vi "_RT_CtrlLoop_Pub_Wfm_ProcessCodes.vi"(7 "Function":T1, 8 "error in (no error)":errorcluster, 10 "EventCodes_U64Arr in":u64[](array[numeric])) -> (0 "error out":errorcluster, 1 "SigLength out":i32, 2 "EventCodes_U64Arr out":u64[](array[numeric]), 4 "DynamicTimeout":i32)   [LabVIEW 2018]
uses:
  Ctl/_ctl_Integrated_Cmd.ctl
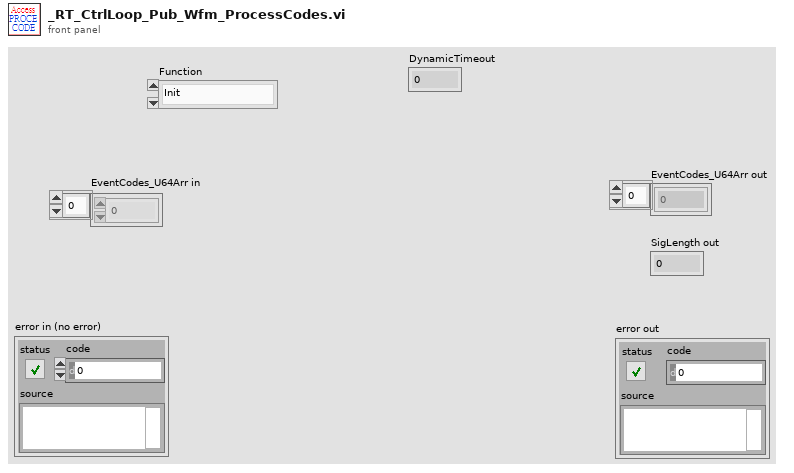
[diagram p1: front panel]
types:
  T1 = typedef "_ctl_Integrated_Cmd.ctl" = enum8{"Init", "Set", "Get", "Read", "Write", "Send", "Idle", "Startup", "Execution", "End", "Close"}
  T2 = enum16{"open", "replace", "create", "open or create", "replace or create", "replace or create with confirmation"}
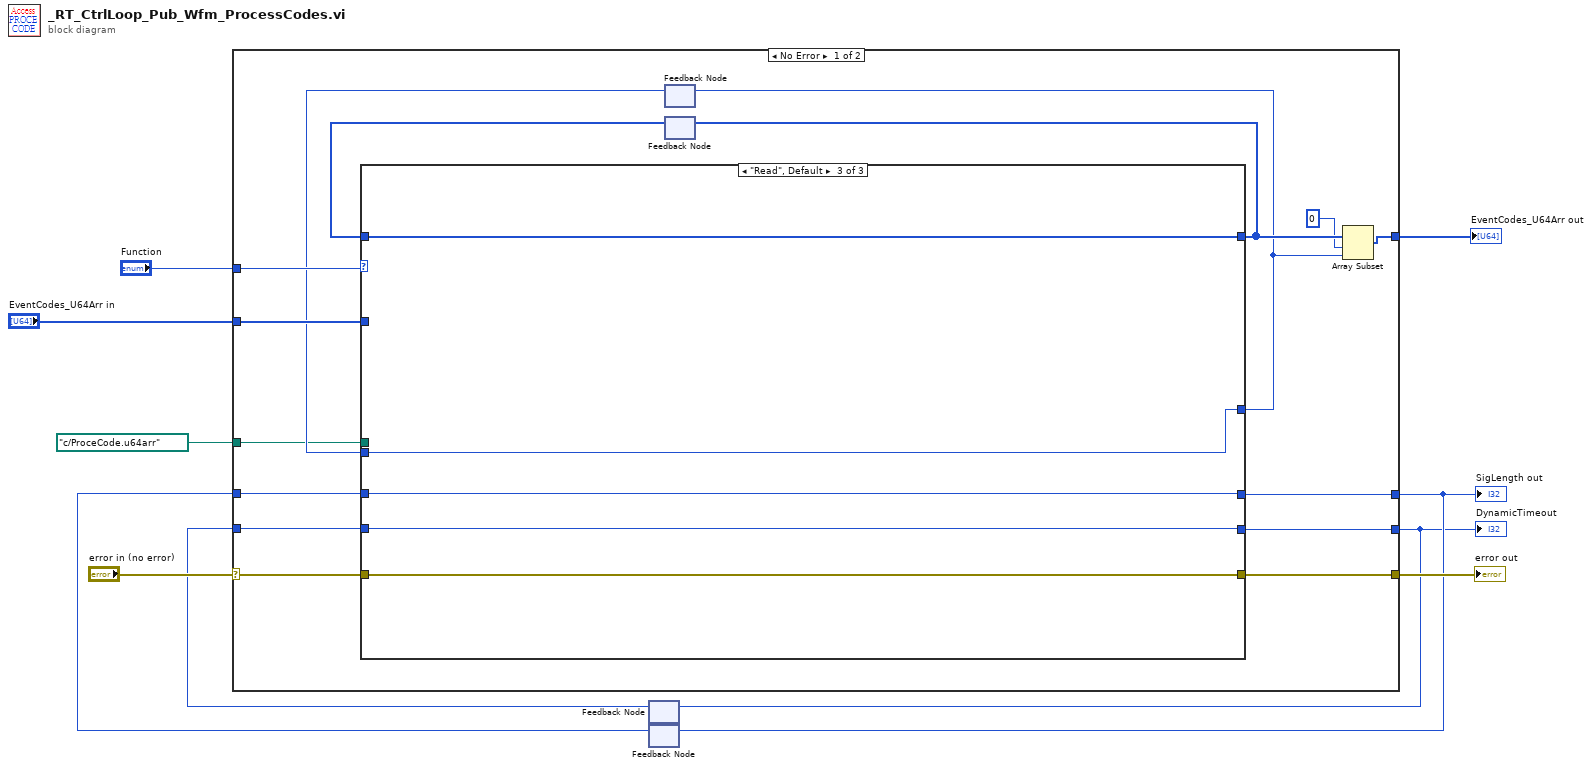
[diagram p0: block diagram]
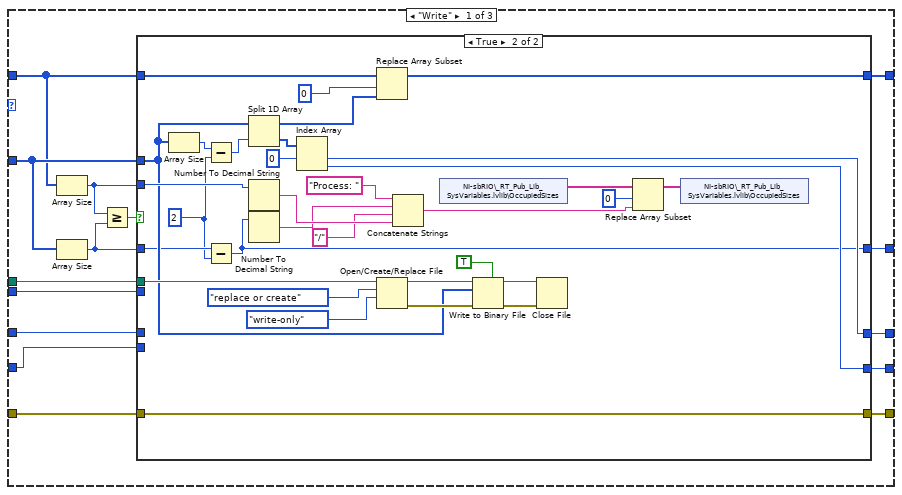
[diagram p2: hidden frame]
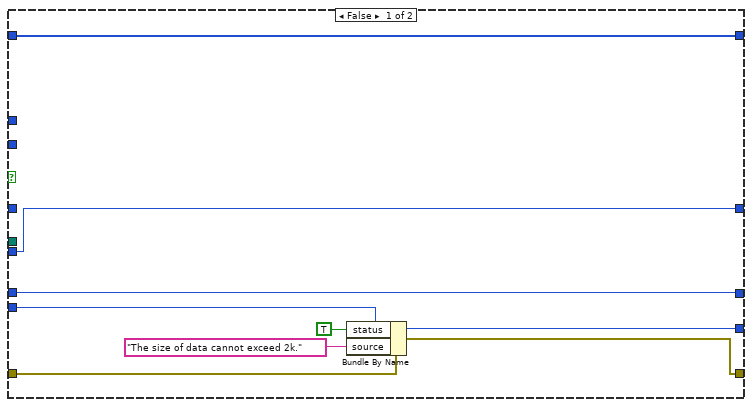
[diagram p3: hidden frame]
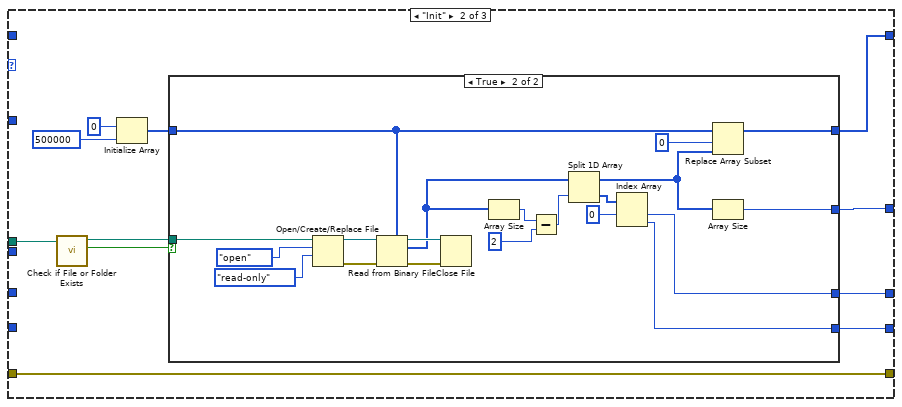
[diagram p4: hidden frame]
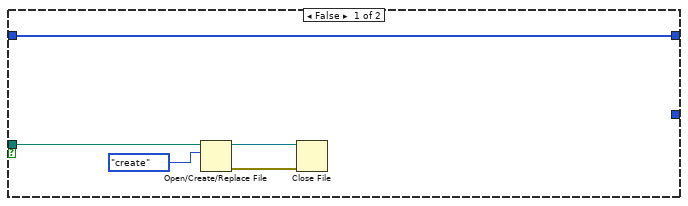
[diagram p5: hidden frame]
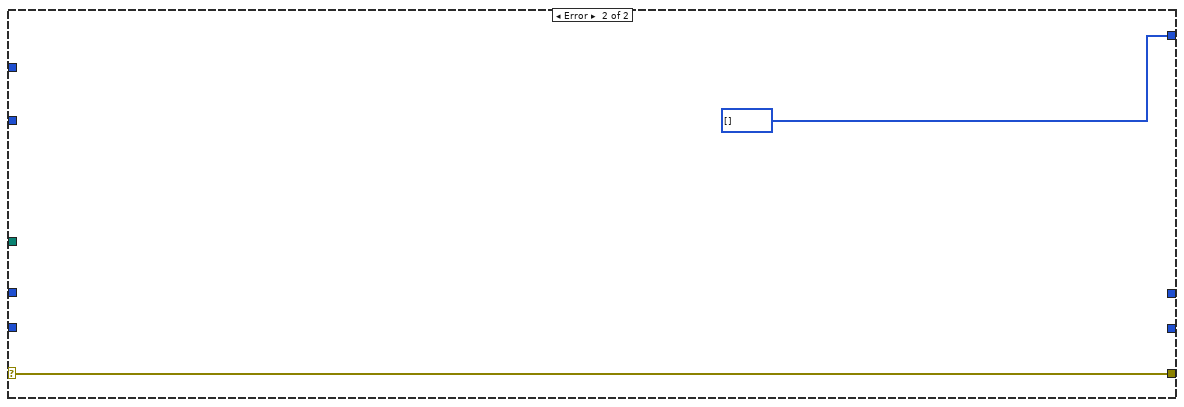
[diagram p6: hidden frame]
diagram:
  n1 = feedback #1() -> (w2:u64)  [unwired: 1 in]
  n2 = feedback #2() -> (w4:u64)  [unwired: 1 in]
  n3 = case shown="No Error" "error in (no error)" {
    selector: "error in (no error)" -> [w22 w123]
    tunnel: "Function" -> [w25 _]
    tunnel: "EventCodes_U64Arr in" -> [w24 _]
    tunnel: [w21 w123] -> w8
    tunnel: [w16 u64[] []] -> w7
    tunnel: w4 -> [w14 _]
    tunnel: [w15 _] -> w5
    tunnel: path "c:/ProceCode.u64arr" ("file path (use dialog)") -> [w13 _]
    tunnel: [w12 _] -> w1
    tunnel: w2 -> [w11 _]
    frame No Error {
      n4 = feedback #3() -> (w20:i32)  [unwired: 1 in]
      n5 = feedback #4() -> (w23:u64[])  [unwired: 1 in]
      n6 = case shown="\"Read\", Default" w25 {
        tunnel: w24 -> [w39 _ _]
        tunnel: [w40 w86 w121] -> w19
        tunnel: w23 -> [w37 _ w121]
        tunnel: w22 -> [w36 w89 w120]
        tunnel: [w35 w89 w120] -> w21
        tunnel: [w33 w85 w119] -> w18
        tunnel: w20 -> [w32 _ w119]
        tunnel: [w30 w83 w118] -> w15
        tunnel: w14 -> [w29 _ w118]
        tunnel: w13 -> [w28 w84 _]
        tunnel: [w27 w82 w117] -> w12
        tunnel: w11 -> [w26 _ w117]
        frame "Write" {
          n7 = Array Size(array=w37) -> (size(s)=w31:i32)
          n8 = Array Size(array=w39) -> (size(s)=w34:i32)
          n9 = Greater Or Equal?(x=w31, y=w34) -> (x >= y?=w38:bool)
          n10 = case shown="True" w38 {
            tunnel: w37 -> [w48 w80]
            tunnel: [w48 w79] -> w40
            tunnel: w39 -> [_ w54]
            tunnel: w36 -> [w47 w77]
            tunnel: [w44 w77] -> w35
            tunnel: w34 -> [_ w51]
            tunnel: [w43 w50] -> w33
            tunnel: w32 -> [w43 _]
            tunnel: w31 -> [_ w69]
            tunnel: [w42 w64] -> w30
            tunnel: w29 -> [w42 _]
            tunnel: w28 -> [_ w62]
            tunnel: [w41 w53] -> w27
            tunnel: w26 -> [w41 _]
            frame False {
              n11 = Bundle By Name(cluster=w47, "status"=TRUE, "source"="The size of data cannot exceed 2k.") -> (w44:errorcluster)
            }
            frame True {
              w49 = 2 ("x")
              n12 = Array Size(array=w54) -> (size(s)=w67:i32)
              n13 = Subtract(x=w67, y=w49) -> (x-y=w68:i32)
              n14 = Subtract(x=w51, y=w49) -> (x-y=w50:i32)
              n15 = Split 1D Array(array=w54, index=w68) -> (first subarray=w57:u64[], second subarray=w66:u64[])
              n16 = Number To Decimal String(number=w69) -> (decimal integer string=w73:string)  [unwired: 1 in]
              n17 = Number To Decimal String(number=w50) -> (decimal integer string=w72:string)  [unwired: 1 in]
              n18 = Index Array(array=w66, index #1=0 ("index")) -> (element #1=w64:u64, element #2=w53:u64)  [unwired: 1 in]
              n19 = Replace Array Subset(array=w80, new element=w57, index=0) -> (w79:u64[])
              n20 = Open/Create/Replace File(file path (use dialog)=w62, operation (0:open)=T2."replace or create", access (0:read/write)=enum16{"read/write", "read-only", "write-only"}."write-only") -> (refnum out=w60:refnum<file>, error out=w59:errorcluster)  [unwired: 3 in, 1 out]
              n21 = Concatenate Strings("Process: " ("element"), w72, "/" ("element"), w73) -> (w76:string)
              n22 = shared-variable "NI-sbRIO\\_RT_Pub_Lib_SysVariables.lvlib\\OccupiedSizes"() -> (w63:string[])  [unwired: 1 in, 1 out]
              n23 = Write to Binary File(file (use dialog)=w60, data=w54, error in=w59, 5:TRUE ("prepend array or string size? (T)")) -> (refnum out=w56:refnum<file>, error out=w55:errorcluster)  [unwired: 2 in, 1 out]
              n24 = Close File(refnum=w56, error in=w55) -> ()  [unwired: 2 out]
              n25 = Replace Array Subset(array=w63, new element=w76, index=0) -> (w74:string[])
              n26 = shared-variable "NI-sbRIO\\_RT_Pub_Lib_SysVariables.lvlib\\OccupiedSizes"(w74) -> ()  [unwired: 1 in, 1 out]
            }
          }
        }
        frame "Init" {
          n27 = call <vilib>:"Check if File or Folder Exists.vi"("path"=w84) -> ("file or folder exists?"=w81:bool, "dup path"=w88:path)  [unwired: 8 in, 1 out]
          n28 = Initialize Array(u64 0, 500000 ("dimension size")) -> (w87:u64[])
          n29 = case shown="True" w81 {
            tunnel: w88 -> [w95 w113]
            tunnel: w87 -> [w96 w97]
            tunnel: [w96 w108] -> w86
            tunnel: [_ w107] -> w85
            tunnel: [_ w103] -> w83
            tunnel: [_ w99] -> w82
            frame False {
              n30 = Open/Create/Replace File(file path (use dialog)=w95, operation (0:open)=T2."create") -> (refnum out=w93:refnum<file>, error out=w92:errorcluster)  [unwired: 4 in, 1 out]
              n31 = Close File(refnum=w93, error in=w92) -> ()  [unwired: 2 out]
            }
            frame True {
              n32 = Open/Create/Replace File(file path (use dialog)=w113, operation (0:open)=T2."open", access (0:read/write)=enum16{"read/write", "read-only", "write-only"}."read-only") -> (refnum out=w115:refnum<file>, error out=w114:errorcluster)  [unwired: 3 in, 1 out]
              n33 = Read from Binary File(5:w97, 8:w114, 11:w115) -> (0:w110:errorcluster, 2:w98:u64[], 3:w111:refnum<file>)  [unwired: 3 in, 1 out]
              n34 = Close File(refnum=w111, error in=w110) -> ()  [unwired: 2 out]
              n35 = Array Size(array=w98) -> (size(s)=w101:i32)
              n36 = Subtract(x=w101, y=2) -> (x-y=w106:i32)
              n37 = Split 1D Array(array=w98, index=w106) -> (first subarray=w102:u64[], second subarray=w105:u64[])
              n38 = Index Array(array=w105, index #1=0 ("index")) -> (element #1=w103:u64, element #2=w99:u64)  [unwired: 1 in]
              n39 = Replace Array Subset(array=w97, new element=w102, index=0) -> (w108:u64[])
              n40 = Array Size(array=w102) -> (size(s)=w107:i32)
            }
          }
        }
        frame "Read", Default {
        }
      }
      n41 = feedback-in #3(w18) -> ()
      n42 = feedback-in #4(w19) -> ()
      n43 = Array Subset(array=w19, index=0, length=w18) -> (w16:u64[])
    }
    frame Error {
    }
  }
  "error out" <- w8
  "EventCodes_U64Arr out" <- w7
  "SigLength out" <- w5
  "DynamicTimeout" <- w1
  n44 = feedback-in #1(w1) -> ()
  n45 = feedback-in #2(w5) -> ()
